vi "combineCommandFrame.vi"(1 "Address":string="AAAAAAAAAAAA", 2 "DataSection":string, 3 "ControlCode":string) -> (0 "ApplicationLayerCommand":string)   [LabVIEW 2010]
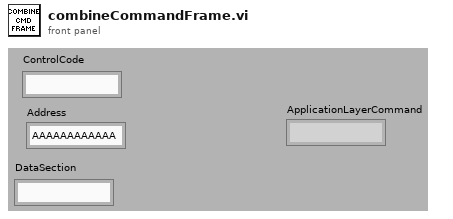
[diagram p1: front panel]
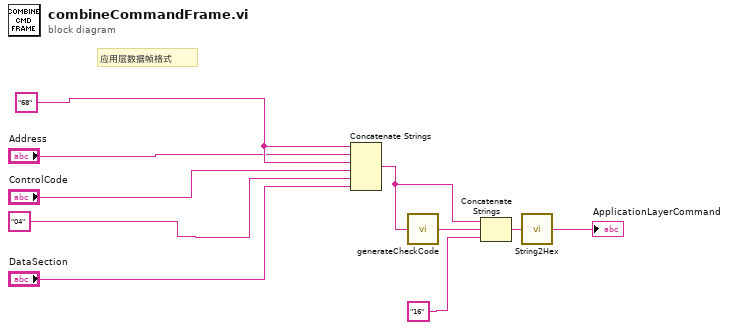
[diagram p0: block diagram]
diagram:
  w4 = "68" ("string")
  # "应用层数据帧格式"
  n1 = Concatenate Strings(w4, "Address", w4, "ControlCode", "04" ("string"), "DataSection") -> (w8:string)
  n2 = call "generateCheckCode.vi"("Data"=w8) -> ("CheckCode"=w7:string)
  n3 = Concatenate Strings(w8, w7, "16" ("string")) -> (w6:string)
  n4 = call "String2Hex.vi"("value"=w6) -> ("String"=→"ApplicationLayerCommand":string)
